vi "create.vi"(10 "reference to close":T1, 11 "original reporter":refnum<class "results reporter.lvclass">) -> (3 "close reference and report out":refnum<class "close reference and report.lvclass">)   [LabVIEW 2013, in "close reference and report.lvclass"]
uses:
  close reference and report.lvclass
  results reporter/results reporter.lvclass
  function definition.ctl
  task token/null task token.lvclass
  close reference and report.lvclass/close reference and report.ctl
  call by reference action.lvclass
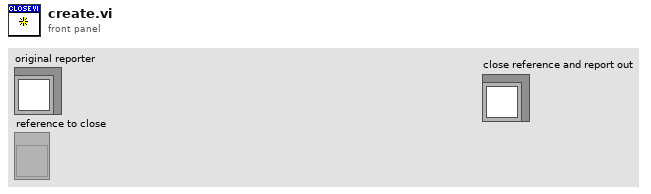
[diagram p1: front panel]
types:
  T1 = typedef "call by reference action.lvclass/function definition.ctl" = refnum<vi>
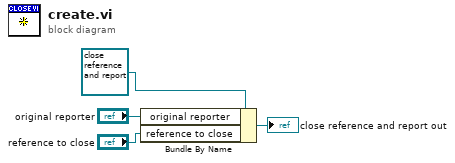
[diagram p0: block diagram]
diagram:
  n1 = Bundle By Name(cluster=refnum<class "close reference and report.lvclass"> refnum ("close reference and report in"), "original reporter"="original reporter", "reference to close"="reference to close") -> (→"close reference and report out":refnum<class "close reference and report.lvclass">)
